vi "DAQ_Test - IO.vi"() -> ()   [LabVIEW 2020]
uses:
  <instrlib>/Keysight DAQ970/Keysight DAQ970.lvlib
panel:
  out "instrument handle out":refnum<k15>
  in  "error in":errorcluster {"code" format="%.0x"}
  out "error out":errorcluster {"code" format="%.0x"}
  in  "VISA resource name":refnum<visa-resource-name>="E000-2600-01"
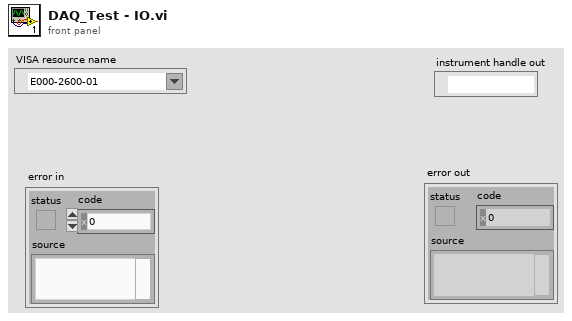
[diagram p1: front panel]
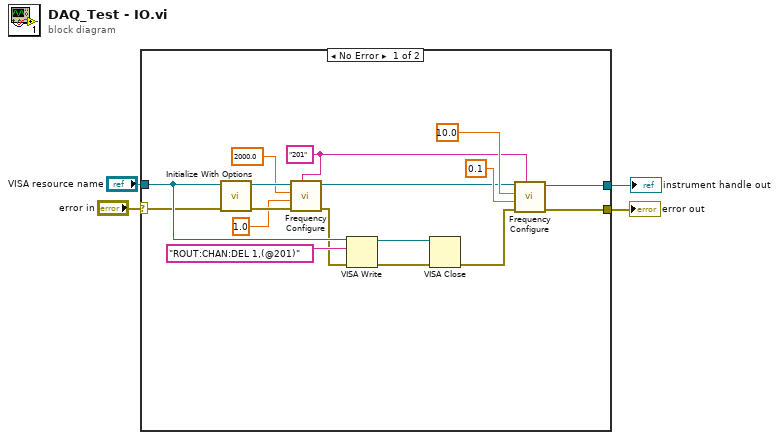
[diagram p0: block diagram]
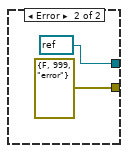
[diagram p2: hidden frame]
diagram:
  n1 = case shown="No Error" "error in" {
    selector: "error in" -> [w5 _]
    tunnel: "VISA resource name" -> [w20 _]
    tunnel: [w8 errorcluster {"status"=FALSE, "code"=999, "source"="error"} ("error out")] -> w3
    tunnel: [w6 refnum<k15> refnum ("instrument handle out")] -> w2
    frame No Error {
      w10 = "201" ("ChannelList")
      n2 = call <instrlib>:"Initialize With Options.vi"("error in (no error)"=w5, "resource string"=w20) -> ("error out"=w18:errorcluster, "instrument handle out"=w17:refnum<k15>)  [unwired: 8 in]
      n3 = call <instrlib>:"Frequency Configure.vi"("ChannelList"=w10, "error in (no error)"=w18, "Resolution"=1.0, "Range"=2000.0, "instrument handle"=w17) -> ("error out"=w15:errorcluster, "instrument handle out"=w7:refnum<k15>)  [unwired: 5 in]
      n4 = VISA Write(VISA resource name=w20, write buffer="ROUT:CHAN:DEL 1,(@201)", error in (no error)=w15) -> (VISA resource name out=w19:refnum<visa-resource-name>, error out=w14:errorcluster)  [unwired: 1 out]
      n5 = VISA Close(VISA resource name=w19, error in (no error)=w14) -> (error out=w9:errorcluster)
      n6 = call <instrlib>:"Frequency Configure.vi"("ChannelList"=w10, "error in (no error)"=w9, "Resolution"=0.1, "Range"=10.0, "instrument handle"=w7) -> ("error out"=w8:errorcluster, "instrument handle out"=w6:refnum<k15>)  [unwired: 5 in]
    }
    frame Error {
    }
  }
  "error out" <- w3
  "instrument handle out" <- w2
